vi "asynchronous output.vi"(9 "Module Info In":T1, 11 "Engine Tags In":T5) -> (1 "Module Info Out":T1, 3 "Engine Tags Out":T5)   [LabVIEW 2013, in "async executor.lvlib"]
doc: "This VI exchanges data with the output method of any asynchronously running modules specified using the 'Output Method Indices' if the 'Execute?' flag for the method is TRUE. It also exchanges the data necessary for that method with the data in the main engine tags. Any errors that occur are stored to be handled at the end of the engine's execution."
uses:
  async executor/async executor.lvlib
  <vilib>/NI/Tag Bus/table/data table.ctl
  async execution info.ctl
  asynchronous process data.ctl
  async command notification.ctl
  <vilib>/NI/Tag Bus Module Framework/runtime/execution settings.ctl
  async error info.ctl
  <vilib>/NI/Tag Bus Module Framework/runtime/error classification.ctl
  Data Table with Transfer Spec.ctl
  <vilib>/NI/Tag Bus/table/transfer specification.ctl
  <vilib>/NI/Tag Bus/tag/Data Type.ctl
  Configuration/Module Decimation.ctl
  Configuration/Module Error Configuration.ctl
  Configuration/Error Actions By Category.ctl
  Configuration/Error Actions.ctl
  <vilib>/NI/Tag Bus/table/data table.lvlib
  <vilib>/NI/Tag Bus/tag/tag descriptor.lvclass
  Configuration/Standard Engine Configuration.lvclass
  <vilib>/NI/Tag Bus Module Framework/runtime/TBM module execution interface.lvclass
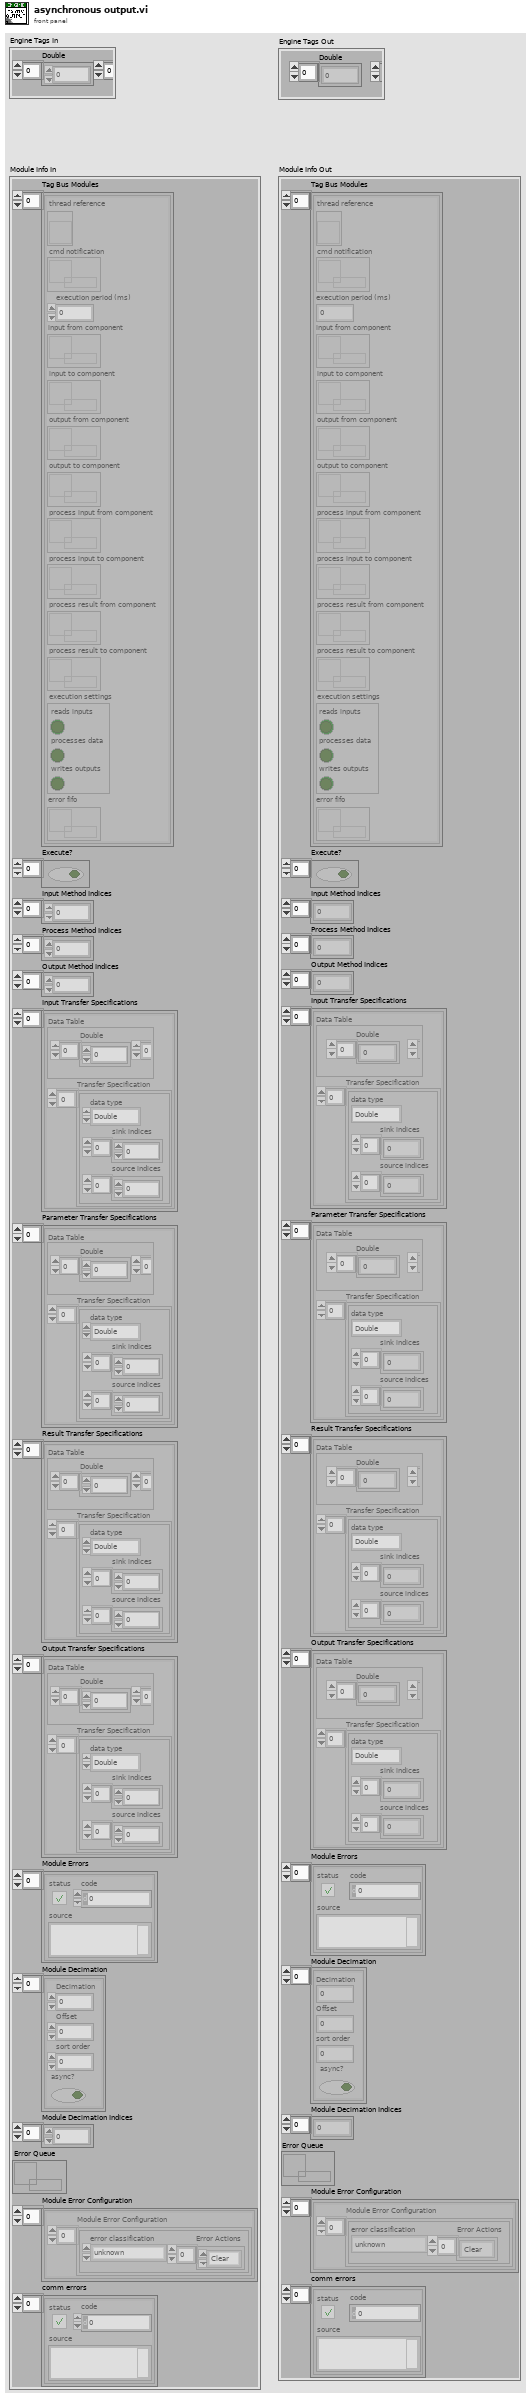
[diagram p1: front panel]
types:
  T1 = typedef "async executor.lvlib/async execution info.ctl" = cluster{"Tag Bus Modules":T2[], "Execute?":bool[], "Input Method Indices":i32[], "Process Method Indices":i32[], "Output Method Indices":i32[], "Input Transfer Specifications":T4[], "Parameter Transfer Specifications":T4[], "Result Transfer Specifications":T4[], "Output Transfer Specifications":T4[], "Module Errors":errorcluster[], "Module Decimation":T8[], "Module Decimation Indices":i32[], "Error Queue":refnum<queue>, "Module Error Configuration":T9[], "comm errors":errorcluster[]}
  T2 = typedef "async executor.lvlib/asynchronous process data.ctl" = cluster{"thread reference":refnum<vi>, "cmd notification":refnum<k33>, "execution period (ms)":i32, "input from component":refnum<queue>, "input to component":refnum<queue>, "output from component":refnum<queue>, "output to component":refnum<queue>, "process input from component":refnum<queue>, "process input to component":refnum<queue>, "process result from component":refnum<queue>, "process result to component":refnum<queue>, "execution settings":T3, "error fifo":refnum<k33>}
  T3 = typedef "TBM module execution interface.lvclass/execution settings.ctl" = cluster{"reads inputs":bool, "processes data":bool, "writes outputs":bool}
  T4 = typedef "Data Table with Transfer Spec.ctl" = cluster{"Data Table":T5, "Transfer Specification":T6[]}
  T5 = typedef "tag bus.lvlib/data table.lvlib/data table.ctl" = cluster{"Double":dbl[], "Single":sgl[], "I64":i64[], "I32":i32[], "I16":i16[], "I8":i8[], "U64":u64[], "U32":u32[], "U16":u16[], "U8":u8[], "Boolean":bool[], "String":string[], "Array of Double":cluster{"DBL Array":dbl[]}[], "Array of Single":cluster{"SGL Array":sgl[]}[], "Array of I64":cluster{"I64 Array":i64[]}[], "Array of I32":cluster{"I32 Array":i32[]}[], "Array of I16":cluster{"I16 Array":i16[]}[], "Array of I8":cluster{"I8 Array":i8[]}[], "Array of U64":cluster{"U64 Array":u64[]}[], "Array of U32":cluster{"U32 Array":u32[]}[], "Array of U16":cluster{"U16 Array":u16[]}[], "Array of U8":cluster{"U8 Array":u8[]}[], "Array of Boolean":cluster{"Boolean Array":bool[]}[], "Array of String":cluster{"String Array":string[]}[]}
  T6 = typedef "tag bus.lvlib/data table.lvlib/transfer specification.ctl" = cluster{"data type":T7, "sink indices":i32[], "source indices":i32[]}
  T7 = typedef "tag bus.lvlib/tag descriptor.lvclass/Data Type.ctl" = enum16{"Double", "Single", "I64", "I32", "I16", "I8", "U64", "U32", "U16", "U8", "Boolean", "String", "Array of Double", "Array of Single", "Array of I64", "Array of I32", "Array of I16", "Array of I8", "Array of U64", "Array of U32", "Array of U16", "Array of U8", "Array of Boolean", "Array of String"}
  T8 = typedef "Standard Engine Configuration.lvclass/Module Decimation.ctl" = cluster{"Decimation":u16, "Offset":u16, "sort order":i32, "async?":bool}
  T9 = typedef "Standard Engine Configuration.lvclass/Module Error Configuration.ctl" = cluster{"Module Error Configuration":T10[]}
  T10 = typedef "Standard Engine Configuration.lvclass/Error Actions By Category.ctl" = cluster{"error classification":T11, "Error Actions":T12[]}
  T11 = typedef "TBM module execution interface.lvclass/error classification.ctl" = enum16{"unknown", "none", "trivial", "recoverable", "critical"}
  T12 = typedef "Standard Engine Configuration.lvclass/Error Actions.ctl" = enum16{"Clear", "Notify", "Stop Component", "Stop Engine", "Safe State", "Attempt Recovery"}
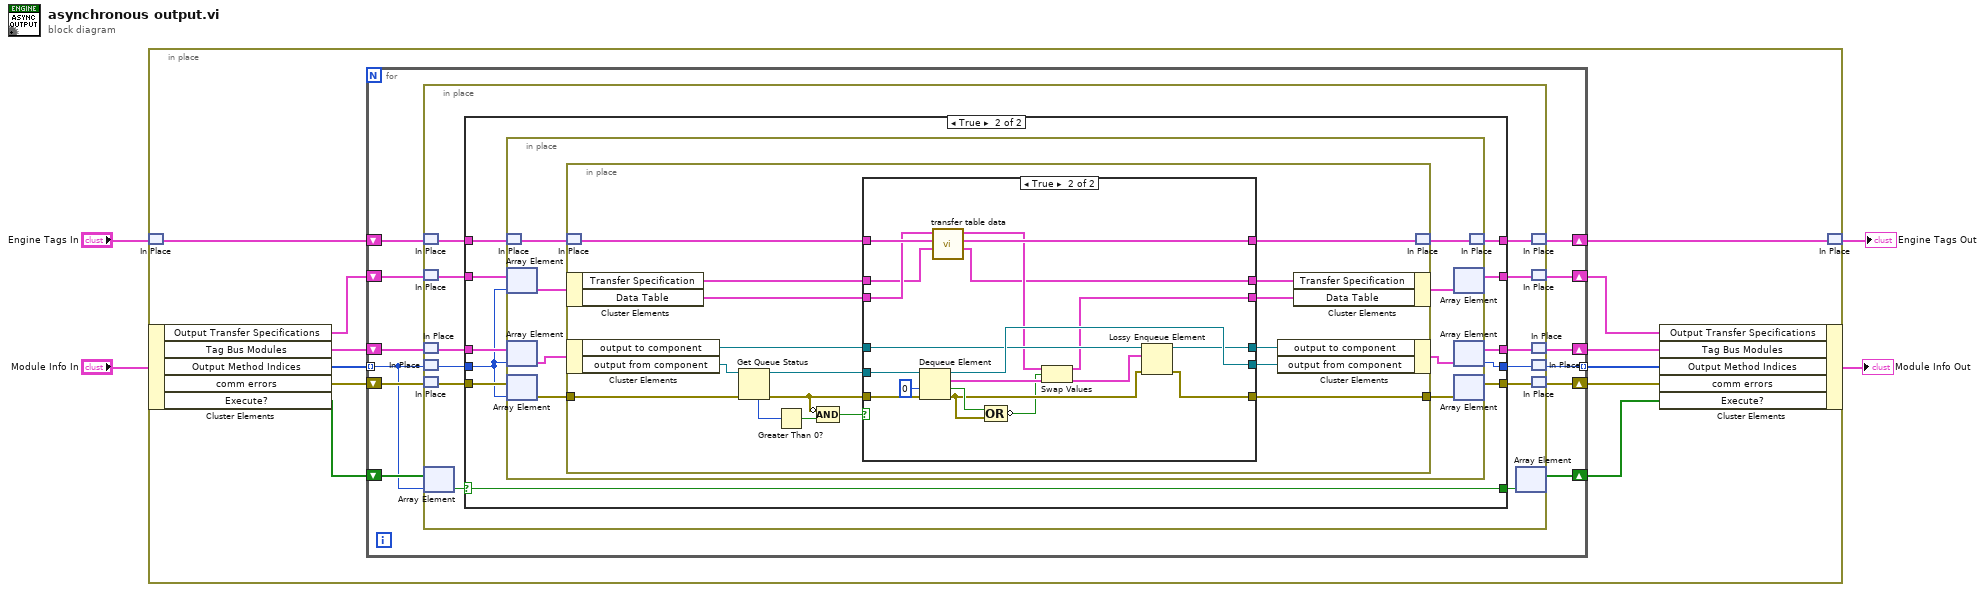
[diagram p0: block diagram]
diagram:
  n1 = in-place {
    n2 = in-place-match #1("Engine Tags In") -> (w15:T5)
    n3 = in-place-cluster #2("Module Info In") -> ("Output Transfer Specifications"=w13:T4[], "Tag Bus Modules"=w10:T2[], "Output Method Indices"=w16:i32[], "comm errors"=w12:errorcluster[], "Execute?"=w6:bool[])
    n4 = for {
      shift-right: [w21] -> w9
      shift-left: w10 -> [w22]
      tunnel: w16 -> [w18] mode=indexing
      shift-right: [w25] -> w14
      shift-left: w15 -> [w26]
      shift-right: [w23] -> w11
      shift-left: w13 -> [w24]
      shift-right: [w19] -> w8
      shift-left: w12 -> [w20]
      tunnel: [w17] -> w7 mode=indexing
      shift-right: [w27] -> w5
      shift-left: w6 -> [w28]
      n5 = in-place {
        n6 = in-place-match #3(w26) -> (w38:T5)
        n7 = in-place-match #4(w24) -> (w36:T4[])
        n8 = in-place-match #5(w22) -> (w34:T2[])
        n9 = in-place-match #6(w18) -> (w30:i32)
        n10 = in-place-match #7(w20) -> (w32:errorcluster[])
        n11 = in-place-array #8(w28, w18) -> (w40:bool)
        n12 = case shown="True" w40 {
          selector: w40 -> [w41 w47]
          tunnel: w38 -> [w46 w57]
          tunnel: [w46 w56] -> w37
          tunnel: w36 -> [w45 w55]
          tunnel: w34 -> [w44 w54]
          tunnel: w32 -> [w42 w53]
          tunnel: [w45 w52] -> w35
          tunnel: [w42 w51] -> w31
          tunnel: [w44 w50] -> w33
          tunnel: w30 -> [w43 w49]
          tunnel: [w43 w48] -> w29
          tunnel: [w41 w47] -> w39
          frame False {
          }
          frame True {
            n13 = in-place {
              n14 = in-place-match #9(w57) -> (w65:T5)
              n15 = in-place-array #10(w55, w49) -> (w63:T4)
              n16 = in-place-array #11(w54, w49) -> (w61:T2)
              n17 = in-place-array #12(w53, w49) -> (w59:errorcluster)
              n18 = in-place {
                in-place-border: w59 -> [w77]
                in-place-border: [w72] -> w58
                n19 = in-place-match #13(w65) -> (w82:T5)
                n20 = in-place-cluster #14(w63) -> ("Transfer Specification"=w79:T6[], "Data Table"=w75:T5)
                n21 = in-place-cluster #15(w61) -> ("output to component"=w74:refnum<queue>, "output from component"=w71:refnum<queue>)
                n22 = Get Queue Status(queue=w71, error in (no error)=w77) -> (queue out=w70:refnum<queue>, error out=w66:errorcluster, # elements in queue=w69:i32)  [unwired: 1 in, 5 out]
                n23 = Greater Than 0?(x=w69) -> (x > 0?=w68:bool)
                n24 = Compound Arithmetic op=AND(invert w66, w68) -> (w67:bool)
                n25 = case shown="True" w67 {
                  tunnel: w82 -> [w83 w94]
                  tunnel: [w83 w93] -> w81
                  tunnel: [w85 w97] -> w80
                  tunnel: w79 -> [w84 w90]
                  tunnel: [w84 w89] -> w78
                  tunnel: [w88 w105] -> w76
                  tunnel: w75 -> [w85 w92]
                  tunnel: w74 -> [w87 w102]
                  tunnel: [w87 w101] -> w73
                  tunnel: [w86 w100] -> w72
                  tunnel: w70 -> [w88 w99]
                  tunnel: w66 -> [w86 w98]
                  frame False {
                  }
                  frame True {
                    n26 = Dequeue Element(queue=w99, timeout in ms (-1)=0, error in (no error)=w98) -> (queue out=w105:refnum<queue>, element=w103:T5, timed out?=w106:bool, error out=w104:errorcluster)
                    n27 = call <vilib>:"transfer table data.vi"("transfer specification in"=w90, "data table source in"=w94, "data table sink in"=w92) -> ("transfer specification out"=w89:T6[], "data table source out"=w93:T5, "data table sink out"=w91:T5)  [unwired: 6 in]
                    n28 = Compound Arithmetic op=OR(w106, w104) -> (invert w95:bool)
                    n29 = Swap Values(12:w91, 13:w95, 14:w103) -> (1:w97:T5, 3:w96:T5)
                    n30 = Lossy Enqueue Element(queue=w102, element=w96, error in (no error)=w104) -> (queue out=w101:refnum<queue>, error out=w100:errorcluster)  [unwired: 2 out]
                  }
                }
                n31 = in-place-cluster #15("output to component"=w73, "output from component"=w76) -> (w60:T2)
                n32 = in-place-cluster #14("Transfer Specification"=w78, "Data Table"=w80) -> (w62:T4)
                n33 = in-place-match #13(w81) -> (w64:T5)
              }
              n34 = in-place-array #10(w62) -> (w52:T4[])  [unwired: 1 out]
              n35 = in-place-array #11(w60) -> (w50:T2[], w48:i32)
              n36 = in-place-array #12(w58) -> (w51:errorcluster[])  [unwired: 1 out]
              n37 = in-place-match #9(w64) -> (w56:T5)
            }
          }
        }
        n38 = in-place-array #8(w39) -> (w27:bool[])  [unwired: 1 out]
        n39 = in-place-match #3(w37) -> (w25:T5)
        n40 = in-place-match #4(w35) -> (w23:T4[])
        n41 = in-place-match #5(w33) -> (w21:T2[])
        n42 = in-place-match #6(w29) -> (w17:i32)
        n43 = in-place-match #7(w31) -> (w19:errorcluster[])
      }
    }
    n44 = in-place-cluster #2("Output Transfer Specifications"=w11, "Tag Bus Modules"=w9, "Output Method Indices"=w7, "comm errors"=w8, "Execute?"=w5) -> (→"Module Info Out":T1)
    n45 = in-place-match #1(w14) -> (→"Engine Tags Out":T5)
  }
